vi "Main.vi"() -> ()   [LabVIEW 2021]
doc: "The myRIO Project template acquires acceleration data from the onboard accelerometer and displays the changes of acceleration values in a waveform chart."
uses:
  <vilib>/myRIO/Instrument Drivers/Onboard IO/AI/typedefs/AI Reference.ctl
  <vilib>/myRIO/Common/Instrument Driver Framework/Utilities/typedefs/myRIO Generic Hardware Reference.ctl
  <vilib>/myRIO/Common/Instrument Driver Framework/Utilities/typedefs/Hardware Version Enum.ctl
  <vilib>/myRIO/Common/Instrument Driver Framework/Utilities/typedefs/myRIO v1.0 Reference.ctl
  <vilib>/myRIO/Common/Instrument Driver Framework/Utilities/typedefs/Generic FPGA Reference.ctl
  <vilib>/myRIO/Common/Instrument Driver Framework/myRIO v1.0/AI/typedefs/AI Channels List.ctl
  <vilib>/myRIO/Common/Instrument Driver Framework/myRIO v1.0/AI/typedefs/AI Channels Enum.ctl
  <vilib>/myRIO/Common/Instrument Driver Framework/Utilities/typedefs/Analog Scaling Constants List.ctl
  <vilib>/myRIO/Common/Instrument Driver Framework/Utilities/typedefs/Analog Scaling Constants.ctl
  <vilib>/userDefined/High Color/nirio_resource_hc.ctl
  <vilib>/myRIO/Common/Instrument Driver Framework/myRIO v1.0/Encoder/typedefs/Encoder Signal Mode.ctl
  <vilib>/myRIO/Instrument Drivers/Onboard IO/Encoder/typedefs/Encoder Reference.ctl
  <vilib>/myRIO/Common/Instrument Driver Framework/myRIO v1.0/Encoder/typedefs/Encoder Channels Enum.ctl
  <vilib>/myRIO/Common/Instrument Driver Framework/myRIO v1.0/Encoder/typedefs/Encoder Configuration v1.0.ctl
  <vilib>/myRIO/Instrument Drivers/Onboard IO/DIO/typedefs/DIO Reference.ctl
  <vilib>/myRIO/Common/Instrument Driver Framework/myRIO v1.0/DIO/typedefs/DIO Channels List.ctl
  <vilib>/myRIO/Common/Instrument Driver Framework/myRIO v1.0/DIO/typedefs/DIO Channels Enum.ctl
  <vilib>/myRIO/Instrument Drivers/Onboard IO/PWM/typedefs/PWM Reference.ctl
  <vilib>/myRIO/Common/Instrument Driver Framework/myRIO v1.0/PWM/typedefs/PWM Channels Enum.ctl
  <vilib>/myRIO/Instrument Drivers/Onboard IO/PWM/typedefs/PWM Configuration.ctl
  <vilib>/myRIO/Common/Instrument Driver Framework/Utilities/vis/Is FPGA Ref Available.vi
  <vilib>/myRIO/Common/Instrument Driver Framework/myRIO v1.0/AI/vis/myRIO v1.1 Open AI.vi
  <vilib>/myRIO/Instrument Drivers/Onboard IO/AI/vis/Read.vi
  <vilib>/myRIO/Common/Instrument Driver Framework/myRIO v1.0/Encoder/vis/myRIO v1.1 Open Encoder.vi
  <vilib>/myRIO/Instrument Drivers/Onboard IO/Encoder/vis/Read.vi
  <vilib>/myRIO/Common/Instrument Driver Framework/myRIO v1.0/DIO/vis/myRIO v1.1 Open DIO.vi
  <vilib>/myRIO/Instrument Drivers/Onboard IO/DIO/vis/Write.vi
  <vilib>/myRIO/Common/Instrument Driver Framework/myRIO v1.0/PWM/vis/myRIO v1.1 Open PWM.vi
  <vilib>/myRIO/Instrument Drivers/Onboard IO/PWM/vis/Set Duty Cycle and Frequency.vi
  <vilib>/myRIO/Common/Instrument Driver Framework/Utilities/vis/Validate Channels.vi
  <vilib>/myRIO/Common/Instrument Driver Framework/myRIO v1.0/AI/vis/myRIO v1.0 Reserve AI.vi
  <vilib>/myRIO/Common/Instrument Driver Framework/myRIO v1.0/Encoder/vis/myRIO v1.0 Reserve Encoder.vi
  <vilib>/myRIO/Common/Instrument Driver Framework/myRIO v1.0/DIO/vis/myRIO v1.0 Reserve DIO.vi
  <vilib>/myRIO/Common/Instrument Driver Framework/myRIO v1.0/PWM/vis/myRIO v1.0 Reserve PWM.vi
  <vilib>/myRIO/Common/Instrument Driver Framework/myRIO v1.0/UART/vis/myRIO v1.0 Close UART.vi
  <vilib>/myRIO/Common/Instrument Driver Framework/myRIO v1.0/AI/vis/myRIO v1.0 Build MUX Configuration AI.vi
  <vilib>/myRIO/Common/Instrument Driver Framework/myRIO v1.0/Resource Manager/vis/myRIO v1.0 Reserve Channel List.vi
  <vilib>/myRIO/Common/Instrument Driver Framework/myRIO v1.0/Encoder/vis/myRIO v1.0 Build MUX Configuration Encoder.vi
  <vilib>/myRIO/Common/Instrument Driver Framework/myRIO v1.0/DIO/vis/myRIO v1.0 Build MUX Configuration DIO.vi
  <vilib>/myRIO/Common/Instrument Driver Framework/myRIO v1.0/PWM/vis/myRIO v1.0 Build MUX Configuration PWM.vi
  <vilib>/myRIO/Common/Instrument Driver Framework/myRIO v1.0/Resource Manager/vis/myRIO v1.0 Reserve Channel.vi
  <vilib>/myRIO/Common/Instrument Driver Framework/myRIO v1.0/Resource Manager/vis/myRIO v1.0 Unreserve Channel.vi
  <vilib>/myRIO/Common/Instrument Driver Framework/myRIO v1.0/Resource Manager/vis/myRIO v1.0 Create Configuration List.vi
  <vilib>/myRIO/Common/Instrument Driver Framework/myRIO v1.0/Resource Manager/vis/myRIO v1.0 Build Mutex Name.vi
  <vilib>/Utility/VariantDataType/GetNumericInfo.vi
  <vilib>/Utility/error.llb/Error Cluster From Error Code.vi
  <vilib>/myRIO/Common/Instrument Driver Framework/myRIO v1.0/myRIO v1.1 Open.vi
  <vilib>/myRIO/Common/Instrument Driver Framework/myRIO v1.0/AI/vis/myRIO v1.0 Get Scaling Constants AI.vi
  <vilib>/myRIO/Common/Instrument Driver Framework/Utilities/vis/IO Manager.vi
  <vilib>/myRIO/Common/Instrument Driver Framework/Utilities/vis/Configuration Manager.vi
  <vilib>/myRIO/Common/Instrument Driver Framework/myRIO v1.0/myRIO v1.0 Close.vi
  <vilib>/myRIO/Common/Instrument Driver Framework/myRIO v1.0/AI/vis/myRIO v1.0 Read AI.vi
  <vilib>/myRIO/Common/Instrument Driver Framework/myRIO v1.0/Resource Manager/vis/myRIO v1.0 Configure IO.vi
  <vilib>/myRIO/Common/Instrument Driver Framework/myRIO v1.0/Encoder/vis/myRIO v1.0 Configure Encoder.vi
  <vilib>/myRIO/Common/Instrument Driver Framework/myRIO v1.0/Encoder/vis/myRIO v1.0 Read Encoder.vi
  <vilib>/addons/Fuzzy Logic/FL Fuzzy Controller (MIMO).vi
  <vilib>/myRIO/Common/Instrument Driver Framework/myRIO v1.0/DIO/vis/myRIO v1.0 Write DIO.vi
  <vilib>/myRIO/Common/Instrument Driver Framework/myRIO v1.0/PWM/vis/myRIO v1.0 Write PWM.vi
  <vilib>/myRIO/Common/Instrument Driver Framework/Utilities/vis/FPGA Ref Manager.vi
  <vilib>/myRIO/Common/Instrument Driver Framework/myRIO v1.0/myRIO v1.0 Reset FPGA.vi
  <vilib>/myRIO/Common/Instrument Driver Framework/myRIO v1.0/IRQ/vis/myRIO v1.0 IRQ Info FGV.vi
  <vilib>/myRIO/Common/Instrument Driver Framework/myRIO v1.0/IRQ/vis/myRIO v1.0 Timer IRQ Info FGV.vi
  <vilib>/myRIO/Common/Instrument Driver Framework/myRIO v1.0/IRQ/vis/myRIO v1.0 ISR Agent.vi
  <vilib>/myRIO/Instrument Drivers/Utilities/vis/Reset Index.vi
  <vilib>/myRIO/Common/Instrument Driver Framework/myRIO v1.0/Resource Manager/vis/myRIO v1.0 Block Write Resource Manager.vi
  <vilib>/myRIO/Express VI/Onboard IO/AI/AI Express VI.xnode
  <vilib>/myRIO/Instrument Drivers/Onboard IO/AI/vis/myRIO AI Open.xnode
  <vilib>/myRIO/Express VI/Onboard IO/Encoder/Encoder Express VI.xnode
  <vilib>/myRIO/Common/Instrument Driver Framework/myRIO v1.0/Encoder/typedefs/Encoder Count Direction Enum.ctl
  <vilib>/myRIO/Instrument Drivers/Onboard IO/Encoder/vis/myRIO Encoder Open.xnode
  <vilib>/myRIO/Express VI/Onboard IO/DO/DO Express VI.xnode
  <vilib>/myRIO/Instrument Drivers/Onboard IO/DIO/vis/myRIO DIO Open.xnode
  <vilib>/myRIO/Express VI/Onboard IO/PWM/PWM Express VI.xnode
  <vilib>/myRIO/Instrument Drivers/Onboard IO/PWM/vis/myRIO PWM Open.xnode
  <vilib>/myRIO/Instrument Drivers/Onboard IO/AI/AI.lvlib
  <vilib>/myRIO/Instrument Drivers/Onboard IO/PWM/PWM.lvlib
  <vilib>/myRIO/Instrument Drivers/Onboard IO/DIO/DIO.lvlib
  <vilib>/myRIO/Instrument Drivers/Onboard IO/Encoder/Encoder.lvlib
  <vilib>/myRIO/Instrument Drivers/Utilities/Utilities.lvlib
  <vilib>/addons/Fuzzy Logic/NI_Fuzzy_Logic_API.lvlib
panel:
  in  "Actuator":bool
  in  "Left Encoder Limit":dbl
  in  "Right Encoder Limit":dbl
  out "Pendulum Angle (Voltage)":dbl(knob) scale=0.0..5.0
  out "Pendulen Angle (Degree)":dbl(knob) scale=-180.0..180.0
  out "Encoder Direction":enum16{"Counting Up", "Counting Down"}(ring)
  out "Overflow":bool
  in  "Reset Counter":bool
  out "Encoder Value":i32
  out "Feedback":dbl format="%#.2g"
  out "Set Point":dbl format="%#.2g"
  out "Error":dbl format="%#.2g"
  in  "Tab Control":enum32{"PID", "Fuzzy"}(tab)
  in  "Kp":dbl
  in  "Ki":dbl
  in  "Kd":dbl
  out "Proportional":dbl format="%#.2g"
  out "Integral":dbl format="%#.2g"
  out "Derivative":dbl format="%#.2g"
  in  "P EN":bool
  in  "I EN":bool
  in  "D EN":bool
  in  "Safety Gap":dbl
  out "PID Waveform Chart":cluster{dbl, dbl, dbl, dbl}(graph)
  out "Fuzzy Waveform Chart":dbl(graph)
  in  "Fuzzy System File Path":path
  out "error out":errorcluster
  in  "Stop":bool
  # "Instructions:\n1. Check the myRIO target IP address in the project and make sure the target IP address is correct. \n2. Run this VI."
  # "Gap between each side of pulley limit"
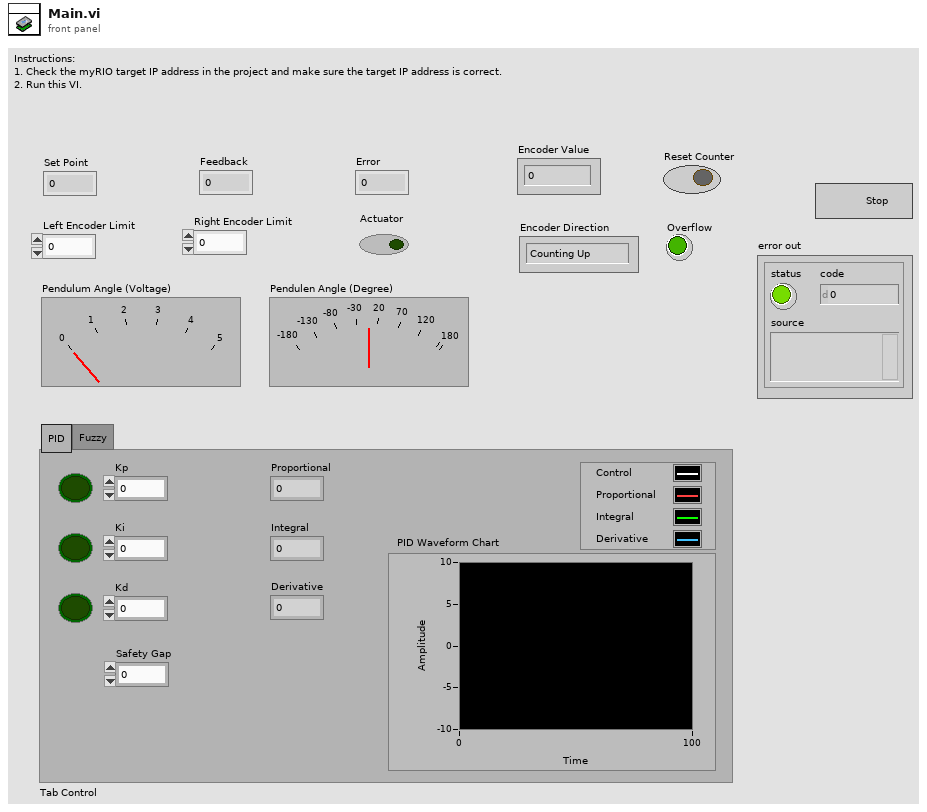
[diagram p1: front panel]
types:
  T1 = typedef "Encoder.lvlib/Encoder Reference.ctl" = cluster{"myRIO Reference":T2, "Encoder Channels Enum":T6}
  T2 = typedef "myRIO Generic Hardware Reference.ctl" = cluster{"myRIO Model":T3, "myRIO Hardware Reference":T4}
  T3 = typedef "Hardware Version Enum.ctl" = enum16{"Unknown", "myRIO-1900", "myRIO-1950", "roboRIO", "NI ELVIS RIO CM", "ELVIS III"}
  T4 = typedef "myRIO v1.0 Reference.ctl" = cluster{"Generic FPGA Reference":T5, "Allow multiple opens":bool}
  T5 = typedef "Generic FPGA Reference.ctl" = refnum<k20>
  T6 = typedef "Encoder Channels Enum.ctl" = enum16{"Not Connected", "C/ENC0", "C/ENC1", "A/ENC", "A/ENC0", "A/ENC1", "A/ENC2", "A/ENC3", "A/ENC4", "A/ENC5", "A/ENC6", "A/ENC7", "A/ENC8", "A/ENC9", "B/ENC", "B/ENC0", "B/ENC1", "B/ENC2", "B/ENC3", "B/ENC4", "B/ENC5", "B/ENC6", "B/ENC7", "B/ENC8", "B/ENC9", "DIO/ENC0", "DIO/ENC1", "DIO/ENC2", "DIO/ENC3", "DIO/ENC4"}
  T7 = typedef "Encoder Signal Mode.ctl" = enum16{"Quadrature phase signal", "Step and direction signal"}
  T8 = typedef "nirio_resource_hc.ctl" = tag
  T9 = typedef "DIO.lvlib/DIO Reference.ctl" = cluster{"myRIO Reference":T2, "DIO Channels List":T10}
  T10 = typedef "DIO Channels List.ctl" = T11[]
  T11 = typedef "DIO Channels Enum.ctl" = enum16{"Not Connected", "C/DIO0", "C/DIO1", "C/DIO2", "C/DIO3", "C/DIO4", "C/DIO5", "C/DIO6", "C/DIO7", "A/DIO0", "A/DIO1", "A/DIO2", "A/DIO3", "A/DIO4", "A/DIO5", "A/DIO6", "A/DIO7", "A/DIO8", "A/DIO9", "A/DIO10", "A/DIO11", "A/DIO12", "A/DIO13", "A/DIO14", "A/DIO15", "A/DIO16", "A/DIO17", "A/DIO18", "A/DIO19", "B/DIO0", "B/DIO1", "B/DIO2", "B/DIO3", "B/DIO4", "B/DIO5", "B/DIO6", "B/DIO7", "B/DIO8", "B/DIO9", "B/DIO10", "B/DIO11", "B/DIO12", "B/DIO13", "B/DIO14", "B/DIO15", "B/DIO16", "B/DIO17", "B/DIO18", "B/DIO19", "LED0", "LED1", "LED2", "LED3", "Button0", "DIO/DIO0", "DIO/DIO1", "DIO/DIO2", "DIO/DIO3", "DIO/DIO4", "DIO/DIO5", "DIO/DIO6", "DIO/DIO7", "DIO/DIO8", "DIO/DIO9", "SPI/CS0", "SPI/CS1", "SPI/CS2", "SPI/CS3", "LED RADIO (Green)", "LED RADIO (Red)", "LED COMM (Green)", "LED COMM (Red)", "LED MODE (Green)", "LED MODE (Red)"}
  T12 = typedef "PWM.lvlib/PWM Reference.ctl" = cluster{"myRIO Reference":T2, "PWM Channels Enum":T13, "PWM Configuration":T14}
  T13 = typedef "PWM Channels Enum.ctl" = enum16{"Not Connected", "C/PWM0", "C/PWM1", "A/PWM0", "A/PWM1", "A/PWM2", "A/PWM3", "A/PWM4", "A/PWM5", "A/PWM6", "A/PWM7", "A/PWM8", "A/PWM9", "A/PWM10", "A/PWM11", "A/PWM12", "A/PWM13", "A/PWM14", "A/PWM15", "A/PWM16", "A/PWM17", "A/PWM18", "A/PWM19", "B/PWM0", "B/PWM1", "B/PWM2", "B/PWM3", "B/PWM4", "B/PWM5", "B/PWM6", "B/PWM7", "B/PWM8", "B/PWM9", "B/PWM10", "B/PWM11", "B/PWM12", "B/PWM13", "B/PWM14", "B/PWM15", "B/PWM16", "B/PWM17", "B/PWM18", "B/PWM19", "PWM/PWM0", "PWM/PWM1", "PWM/PWM2", "PWM/PWM3", "PWM/PWM4", "PWM/PWM5", "PWM/PWM6", "PWM/PWM7", "PWM/PWM8", "PWM/PWM9"}
  T14 = typedef "PWM.lvlib/PWM Configuration.ctl" = cluster{"Frequency":dbl, "Duty Cycle":dbl}
  T15 = typedef "AI.lvlib/AI Reference.ctl" = cluster{"myRIO Reference":T2, "AI Channels List":T16, "AI Scaling Constants List":T18}
  T16 = typedef "AI Channels List.ctl" = T17[]
  T17 = typedef "AI Channels Enum.ctl" = enum16{"Not Connected", "AudioIn/Left", "AudioIn/Right", "C/AI0", "C/AI1", "A/AI0", "A/AI1", "A/AI2", "A/AI3", "A/AI4", "A/AI5", "A/AI6", "A/AI7", "B/AI0", "B/AI1", "B/AI2", "B/AI3", "B/AI4", "B/AI5", "B/AI6", "B/AI7", "AI/AI0", "AI/AI1", "AI/AI2", "AI/AI3", "A/AI0 (DIFF)", "A/AI1 (DIFF)", "A/AI2 (DIFF)", "A/AI3 (DIFF)", "B/AI0 (DIFF)", "B/AI1 (DIFF)", "B/AI2 (DIFF)", "B/AI3 (DIFF)"}
  T18 = typedef "Analog Scaling Constants List.ctl" = T19[]
  T19 = typedef "Analog Scaling Constants.ctl" = cluster{"LSB Weight (Volts)":dbl, "Offset (Volts)":dbl, "Signed?":bool}
  T20 = typedef "Encoder Count Direction Enum.ctl" = enum16{"Counting Up", "Counting Down"}
  T21 = typedef "NI_Fuzzy_Logic_API.lvlib/FL System.ctl" = cluster{"input variables":T22[], "output variables":T22[], "rules":T25[], "defuzzification method":T31, "description":string, "user MF interpolating polynomials":T32[]}
  T22 = typedef "NI_Fuzzy_Logic_API.lvlib/FL Variable.ctl" = cluster{"name":string, "range":dbl[], "MFs":T23[]}
  T23 = typedef "NI_Fuzzy_Logic_API.lvlib/FL Membership Function.ctl" = cluster{"name":string, "shape":T24, "points":dbl[], "color":u32, "user-defined shape index":i32}
  T24 = typedef "NI_Fuzzy_Logic_API.lvlib/FL Membership Function Shape.ctl" = u16
  T25 = typedef "NI_Fuzzy_Logic_API.lvlib/FL Rule.ctl" = cluster{"antecedents":T26[], "antecedent connective":T28, "consequents":T29[], "consequent implication":T30, "degree of support":dbl}
  T26 = typedef "NI_Fuzzy_Logic_API.lvlib/FL Antecedent.ctl" = cluster{"Var Index":i32, "MF Index":i32, "Cond":T27}
  T27 = typedef "NI_Fuzzy_Logic_API.lvlib/FL Modifier.ctl" = u16
  T28 = typedef "NI_Fuzzy_Logic_API.lvlib/FL Antecedent Connective.ctl" = u16
  T29 = typedef "NI_Fuzzy_Logic_API.lvlib/FL Consequent.ctl" = cluster{"Var Index":i32, "MF Index":i32, "Cond":T27}
  T30 = typedef "NI_Fuzzy_Logic_API.lvlib/FL Consequent Implication.ctl" = u16
  T31 = typedef "NI_Fuzzy_Logic_API.lvlib/FL Defuzzification.ctl" = u16
  T32 = typedef "NI_Fuzzy_Logic_API.lvlib/FL Interpolating polynomials.ctl" = cluster{"X":dbl[], "Y":dbl[], "Y(x) coeff":dbl[][], "X(y) coeff":dbl[][], "Area(y) coeff":dbl[][], "coa_x(y) coeff":dbl[][]}
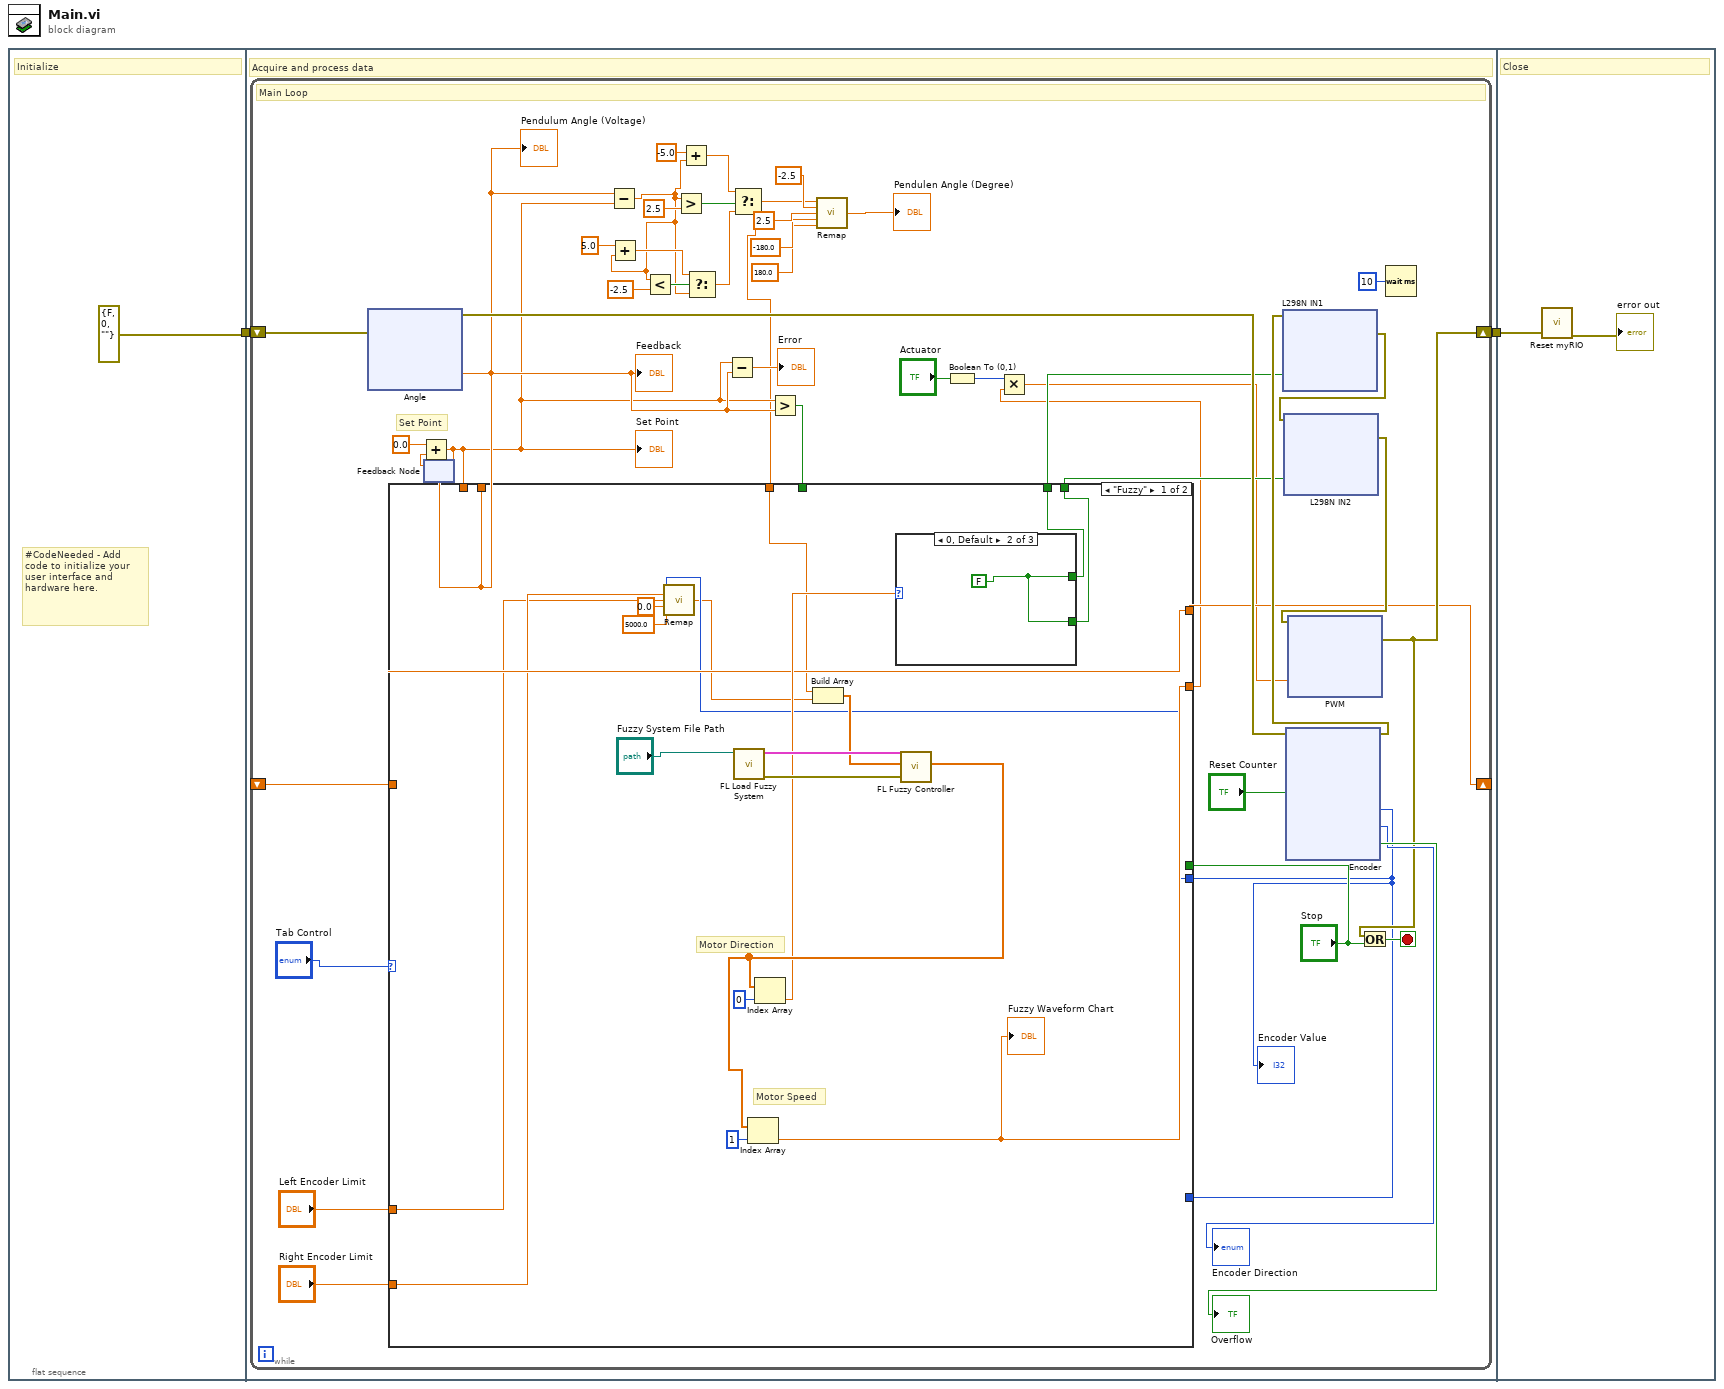
[diagram p0: block diagram]
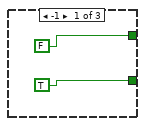
[diagram p2: hidden frame]
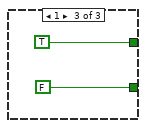
[diagram p3: hidden frame]
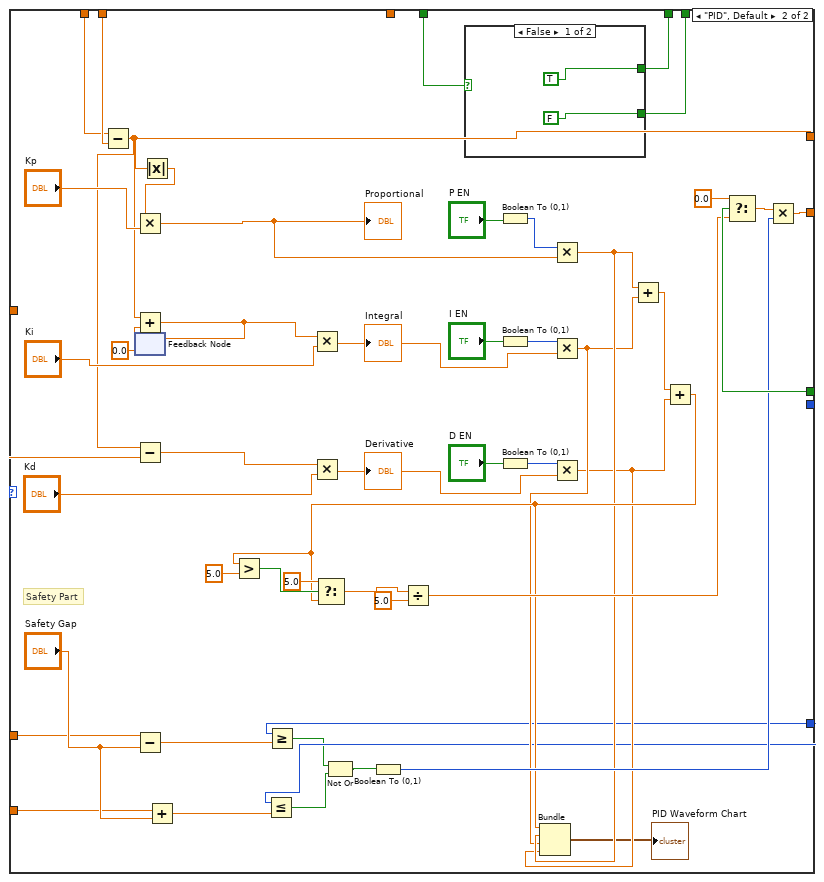
[diagram p4: hidden frame]
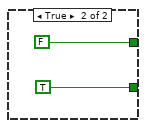
[diagram p5: hidden frame]
diagram:
  n1 = flat-sequence {
    tunnel: [errorcluster {"status"=FALSE, "code"=0, "source"=""} ("error in (no error)")] -> w2
    tunnel: w2 -> [w5]
    tunnel: [w4] -> w1
    tunnel: w1 -> [w319]
    frame #0 {
      # "#CodeNeeded - Add code to initialize your user interface and hardware here."
      # "Initialize"
    }
    frame #1 {
      # "Acquire and process data"
      n2 = while {
        shift-right: [w36] -> w4
        shift-left: w5 -> [w42]
        shift-right: [w32] -> _
        shift-left: _ -> [w49]
        stop <- w51 stop-if-true
        # "Set Point"
        # "Main Loop"
        n3 = xnode "Angle"("error in (no error)"=w42) -> ("A/AI0 (Pin 3)"=w31:dbl, "error out"=w41:errorcluster)
        "Feedback" <- w31
        "Pendulum Angle (Voltage)" <- w31
        n4 = feedback #1(w31) -> (w48:dbl)
        n5 = Add(x=0.0, y=w48) -> (x+y=w30:dbl)
        "Set Point" <- w30
        n6 = feedback-in #1(w30) -> ()
        n7 = Subtract(x=w31, y=w30) -> (x-y=w20:dbl)
        n8 = Add(x=5.0, y=w20) -> (x+y=w22:dbl)
        n9 = Less?(x=w20, y=-2.5) -> (x < y?=w24:bool)
        n10 = Greater?(x=w20, y=2.5) -> (0:w28:bool)
        n11 = Add(x=-5.0, y=w20) -> (x+y=w26:dbl)
        n12 = Select(t=w22, s=w24, f=w20) -> (s? t:f=w25:dbl)
        n13 = Subtract(x=w30, y=w31) -> (x-y=→"Error":dbl)
        n14 = Select(t=w26, s=w28, f=w25) -> (s? t:f=w13:dbl)
        n15 = Greater?(x=w30, y=w31) -> (0:w46:bool)
        n16 = call "Remap.vi"("x"=w13, "In Min"=-2.5, "In Max"=2.5, "Out Min"=-180.0, "Out Max"=180.0) -> ("y"=→"Pendulen Angle (Degree)":dbl)  [unwired: 10 in]
        n17 = Boolean To (0,1)(Boolean="Actuator") -> (0, 1=w9:i16)
        n18 = xnode "Encoder"("Reset Counter"="Reset Counter", "error in (no error)"=w41) -> ("Counter Value"=w12:i32, "Counter Direction"=→"Encoder Direction":T20, "Overflow?"=→"Overflow":bool, "error out"=w40:errorcluster)
        "Encoder Value" <- w12
        n19 = case shown="\"Fuzzy\"" "Tab Control" {
          tunnel: w49 -> [w60 w120]
          tunnel: w46 -> [_ w102]
          tunnel: "Stop" -> [_ w101]
          tunnel: [w62 w98] -> w35
          tunnel: [w63 w97] -> w34
          tunnel: [w60 w95] -> w32
          tunnel: [w59 w90] -> w7
          tunnel: w31 -> [_ w88]
          tunnel: w30 -> [_ w87]
          tunnel: w12 -> [_ w81]
          tunnel: w13 -> [w54 _]
          tunnel: w12 -> [w53 _]
          tunnel: "Right Encoder Limit" -> [w58 w80]
          tunnel: "Left Encoder Limit" -> [w57 w79]
          frame "Fuzzy" {
            # "Motor Speed"
            # "Motor Direction"
            n20 = call "Remap.vi"("x"=w53, "In Min"=w58, "In Max"=w57, "Out Min"=0.0, "Out Max"=5000.0) -> ("y"=w52:dbl)  [unwired: 10 in]
            n21 = call <vilib>:"FL Load Fuzzy System.vi"("file path"="Fuzzy System File Path") -> ("error out"=w69:errorcluster, "fuzzy system out"=w70:T21)  [unwired: 9 in]
            n22 = Build Array(w54, w52) -> (w68:dbl[])
            n23 = call-poly <vilib>:"FL Fuzzy Controller.vi"("error in (no error)"=w69, "input values"=w68, "fuzzy system in"=w70) -> ("output values"=w64:dbl[])  [unwired: 4 in, 4 out]
            n24 = Index Array(array=w64, index=1) -> (element=w59:dbl)
            "Fuzzy Waveform Chart" <- w59
            n25 = Index Array(array=w64, index=0) -> (element=w61:dbl)
            n26 = case shown="0, Default" w61 {
              tunnel: [FALSE w73 TRUE] -> w63
              tunnel: [TRUE w73 FALSE] -> w62
              frame -1 {
              }
              frame 0, Default {
                w73 = FALSE
              }
              frame 1 {
              }
            }
          }
          frame "PID", Default {
            # "Safety Part"
            n27 = Subtract(x=w87, y=w88) -> (x-y=w95:dbl)
            n28 = feedback #2(0.0) -> (w124:dbl)
            n29 = Add(x=w95, y=w124) -> (x+y=w122:dbl)
            n30 = feedback-in #2(w122) -> ()
            n31 = Subtract(x=w95, y=w120) -> (x-y=w118:dbl)
            n32 = Subtract(x=w79, y="Safety Gap") -> (x-y=w94:dbl)
            n33 = Absolute Value(x=w95) -> (abs(x)=w96:dbl)
            n34 = Multiply(x=w96, y="Kp") -> (x*y=w113:dbl)
            "Proportional" <- w113
            n35 = Add(x=w80, y="Safety Gap") -> (x+y=w92:dbl)
            n36 = Less Or Equal?(x=w81, y=w92) -> (x <= y?=w77:bool)
            n37 = Greater Or Equal?(x=w81, y=w94) -> (x >= y?=w76:bool)
            n38 = Multiply(x=w122, y="Ki") -> (x*y=w111:dbl)
            "Integral" <- w111
            n39 = Multiply(x=w118, y="Kd") -> (x*y=w109:dbl)
            "Derivative" <- w109
            n40 = Not Or(1:w77, 2:w76) -> (0:w78:bool)
            n41 = Boolean To (0,1)(Boolean=w78) -> (0, 1=w89:i16)
            n42 = case shown="False" w102 {
              tunnel: [TRUE FALSE] -> w97
              tunnel: [FALSE TRUE] -> w98
              frame False {
              }
              frame True {
              }
            }
            n43 = Boolean To (0,1)(Boolean="P EN") -> (0, 1=w114:i16)
            n44 = Boolean To (0,1)(Boolean="I EN") -> (0, 1=w112:i16)
            n45 = Boolean To (0,1)(Boolean="D EN") -> (0, 1=w110:i16)
            n46 = Multiply(x=w114, y=w113) -> (x*y=w85:dbl)
            n47 = Multiply(x=w112, y=w111) -> (x*y=w84:dbl)
            n48 = Multiply(x=w110, y=w109) -> (x*y=w83:dbl)
            n49 = Add(x=w85, y=w84) -> (x+y=w108:dbl)
            n50 = Add(x=w108, y=w83) -> (x+y=w86:dbl)
            n51 = Greater?(x=w86, y=5.0) -> (0:w106:bool)
            n52 = Select(t=5.0, s=w106, f=w86) -> (s? t:f=w103:dbl)
            n53 = Divide(x=w103, y=5.0) -> (x/y=w99:dbl)
            n54 = Bundle(w86, w85, w84, w83) -> (→"PID Waveform Chart":cluster{dbl, dbl, dbl, dbl})  [unwired: 1 in]
            n55 = Select(t=0.0, s=w101, f=w99) -> (s? t:f=w91:dbl)
            n56 = Multiply(x=w91, y=w89) -> (x*y=w90:dbl)
          }
        }
        n57 = Multiply(x=w9, y=w7) -> (x*y=w6:dbl)
        n58 = xnode "L298N IN1"("A/DIO0 (Pin 11)"=w34, "error in (no error)"=w40) -> ("error out"=w39:errorcluster)
        n59 = xnode "L298N IN2"("A/DIO1 (Pin 13)"=w35, "error in (no error)"=w39) -> ("error out"=w37:errorcluster)
        n60 = xnode "PWM"("Duty Cycle"=w6, "error in (no error)"=w37) -> ("error out"=w36:errorcluster)
        n61 = Or(x=w36, y="Stop") -> (x .or. y?=w51:bool)
        n62 = Wait (ms)(milliseconds to wait=u32 10) -> ()  [unwired: 1 out]
      }
    }
    frame #2 {
      # "Close"
      n63 = call <vilib>:"Reset myRIO.vi"("error in (no error)"=w319) -> ("error out"=→"error out":errorcluster)  [unwired: 10 in]
    }
  }
